vi "getDevices.vi"(1 "Device Class":string="FakeCamSub") -> (0 "All Devices":string[](array[string]))   [LabVIEW 2013]
uses:
  Shared/MySQL/Preset Query Enum.ctl
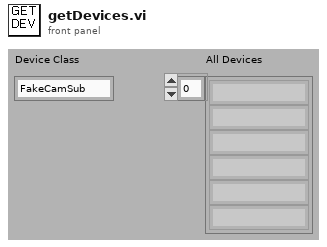
[diagram p1: front panel]
types:
  T1 = typedef "Preset Query Enum.ctl" = enum16{"Get Locations", "Get all IPs and MACs", "Get classes", "Get expt variables to set at scanstart for particular device", "Get expt devices and variables with start values", "Get expt devices and variables (with data to get)", "Get expt devices with data to get", "Get Expt devices and GUIs", "Get all devices basic properties", "Get Virtual Devices Core Info", "Get Expt names", "Get experiment basic properties", "Get experiment alarm variables", "Get MC Ports", "Get device network comm port", "Get devicetype lvclass path", "Get basic device properties", "Get Init Order", "Get all setable variables of a device", "Get device variable aliases", "Get force values of all settable variables", "Get all variables of a devicetype", "Get all variables of a device", "Get plotter details", "Get Saved Scans", "Get Scan Info", "GetGeneralGUIs", "Get expt for plotter", "Get plotter IDs from expt", "Get all devices", "Get all Virtual Devices", "Get all aliases", "Get variable and device info for Virtual Device", "GetItemLocatorIP", "Get IPs for GUIs", "Get DeviceType from Device", "GetLocalPortRange", "GetDevicePresetVariables", "Get Device Configuration", "GetAllPresetNames", "GetAllConfigurationNames", "GetPresetDeviceNames"}
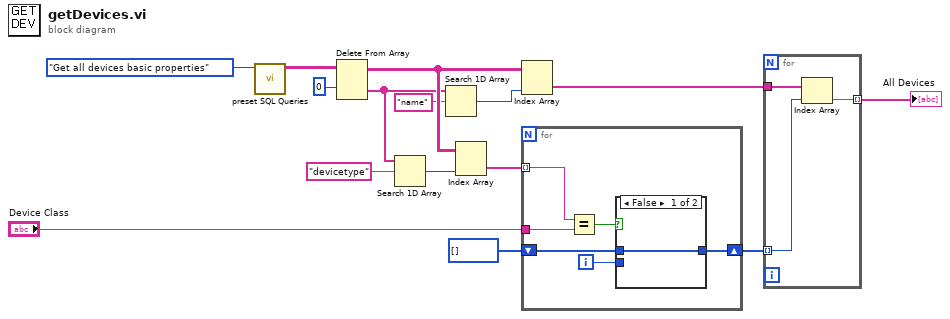
[diagram p0: block diagram]
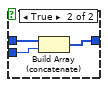
[diagram p2: hidden frame]
diagram:
  n1 = call "preset SQL Queries.vi"("Preset Query"=Preset_Query_Enum."Get all devices basic properties") -> ("data"=w4:string[][])  [unwired: 8 in, 2 out]
  n2 = Delete From Array(array=w4, index (row)=0) -> (deleted portion=w9:string[], array with subset deleted=w11:string[][])  [unwired: 2 in]
  n3 = Search 1D Array(1D array=w9, element="devicetype") -> (index of element=w3:i32)  [unwired: 1 in]
  n4 = Search 1D Array(1D array=w9, element="name") -> (index of element=w12:i32)  [unwired: 1 in]
  n5 = Index Array(array=w11, index (col)=w3) -> (element=w6:string[])  [unwired: 1 in]
  n6 = Index Array(array=w11, index (col)=w12) -> (element=w14:string[])  [unwired: 1 in]
  n7 = for {
    tunnel: w6 -> [w21] mode=indexing
    tunnel: "Device Class" -> [w20]
    shift-right: [w17] -> w13
    shift-left: i32[] [] -> [w16]
    i -> [w18]
    n8 = Equal?(x=w21, y=w20) -> (x = y?=w19:bool)
    n9 = case shown="False" w19 {
      tunnel: w18 -> [_ w25]
      tunnel: [w22 w24] -> w17
      tunnel: w16 -> [w22 w23]
      frame False {
      }
      frame True {
        n10 = Build Array (concatenate)(w23, w25) -> (w24:i32[])
      }
    }
  }
  n11 = for {
    tunnel: w13 -> [w27] mode=indexing
    tunnel: w14 -> [w28]
    tunnel: [w26] -> w15 mode=indexing
    n12 = Index Array(array=w28, index=w27) -> (element=w26:string)
  }
  "All Devices" <- w15
